vi "Read power line frequency.vi"(8 "error in (no error)":errorcluster, 11 "CS++DMM in":refnum<class "CS++DMM.lvclass">) -> (0 "error out":errorcluster, 2 "power line frequency (60.0 Hz)":dbl=60.0 format="%^.2e", 3 "CS++DMM out":refnum<class "CS++DMM.lvclass">)   [LabVIEW 2016, in "CS++DMM.lvlib" / "CS++DMM.lvclass"]
uses:
  CS++DMM.lvclass
  CS++DMM.lvclass/CS++DMM.ctl
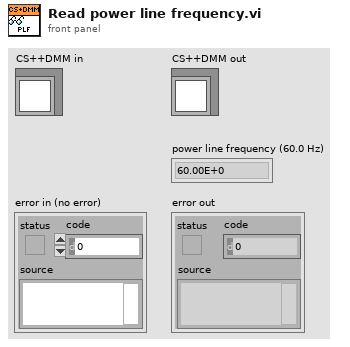
[diagram p1: front panel]
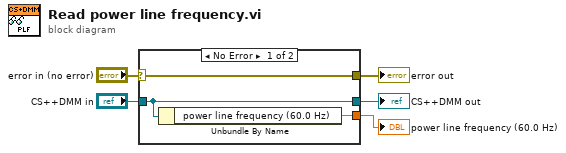
[diagram p0: block diagram]
diagram:
  n1 = case shown="No Error" "error in (no error)" {
    selector: "error in (no error)" -> [w8 w9]
    tunnel: [w8 w9] -> w4
    tunnel: [w7 w10] -> w2
    tunnel: "CS++DMM in" -> [w7 w10]
    tunnel: [w6 _] -> w1
    frame No Error {
      n2 = Unbundle By Name(w7) -> ("power line frequency (60.0 Hz)"=w6:dbl)
    }
    frame Error {
    }
  }
  "error out" <- w4
  "CS++DMM out" <- w2
  "power line frequency (60.0 Hz)" <- w1
